vi "ondas1.vi"() -> ()   [LabVIEW 2018]
uses:
  <vilib>/Analysis/2dsp.llb/2D Real FFT.vi
  <vilib>/Analysis/NI_AALPro.lvlib
panel:
  out "Waveform Chart":dbl[](graph)
  out "Waveform Graph":dbl[](graph)
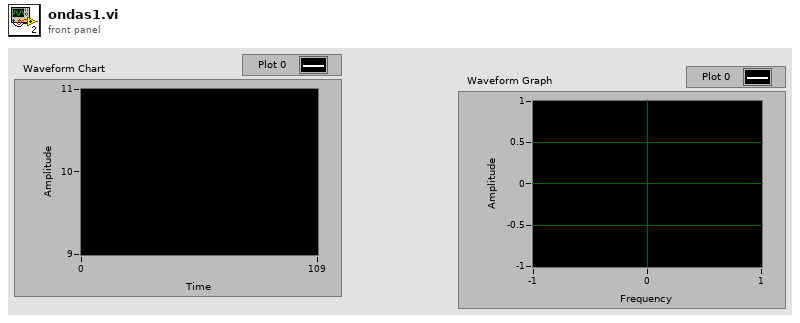
[diagram p1: front panel]
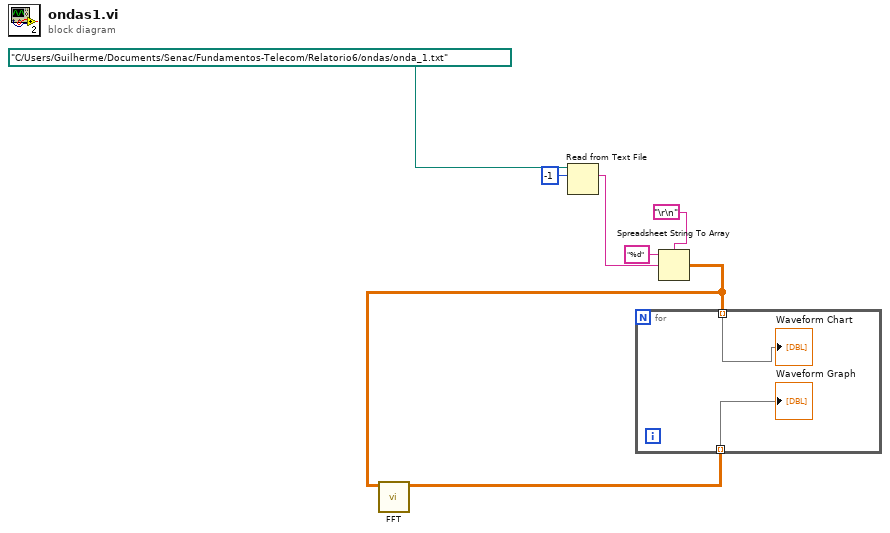
[diagram p0: block diagram]
diagram:
  n1 = Read from Text File(file (use dialog)=path "C:/Users/Guilherme/Documents/Senac/Fundamentos-Telecom/Relatorio6/ondas/onda_1.txt", count=-1) -> (text=w6:string)  [unwired: 2 in, 3 out]
  n2 = Spreadsheet String To Array(delimiter (Tab)="\r\n", format string="%d", spreadsheet string=w6) -> (array=w3:dbl[][])  [unwired: 1 in]
  n3 = call-poly <vilib>:"FFT.vi"("X"=w3) -> ("FFT {X}"=w2:cdb[][])  [unwired: 9 in, 1 out]
  n4 = for {
    tunnel: w3 -> [w9] mode=indexing
    tunnel: w2 -> [w8] mode=indexing
    "Waveform Chart" <- w9
    "Waveform Graph" <- w8
  }
